vi "Set Just Validate.vi"(10 "Just Validate":bool, 11 "CFG JSON Base in":refnum<class "CFG JSON.lvclass">) -> (3 "CFG JSON Base out":refnum<class "CFG JSON.lvclass">)   [LabVIEW 2023, in "HAL GOOP4.lvlib" / "CFG JSON.lvclass"]
uses:
  CFG JSON.lvclass
  CFG JSON.lvclass/CFG JSON.ctl
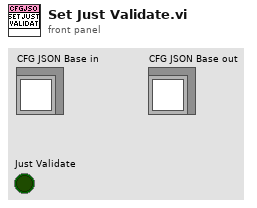
[diagram p1: front panel]
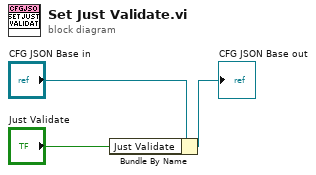
[diagram p0: block diagram]
diagram:
  n1 = Bundle By Name(cluster="CFG JSON Base in", "Just Validate"="Just Validate") -> (→"CFG JSON Base out":refnum<class "CFG JSON.lvclass">)
